vi "Cross_roads.vi"() -> ()   [LabVIEW 2024, in "Road.lvlib"]
uses:
  Road.lvlib
  typedef_GREEN.ctl
  typedef_YELLOW.ctl
  typedef_RED.ctl
  Enum_state.ctl
  typedef_Dane.ctl
  typedef_enum_cykl.ctl
  typedef_Enum_Stan.ctl
  typdef_Timer_Cluster.ctl
  typedef_Time.ctl
  MessageHandler/#typedef_MessageCommand.ctl
  MessageHandler/#typedef_MessageParameters.ctl
  MessageHandler/#typedef_MessageEnum.ctl
  MessageHandler/#typedef_CommunicationModuleAction.ctl
  MessageHandler/#typedef_Message.ctl
  GUI.lvlib
panel:
  in  "Boolean":bool
  out "State_4":bool
  out "Stoper":u32
  out "C3":T1
  out "C2":T1
  out "CC":T2
  out "D3":T3
  out "D2":T3
  out "DD":T4
  out "BBB":T5
  out "AA":T6
  out "A2":T7
  in  "Stop":bool
  out "BB":T5
  out "AAA":T6
  out "CCC":T2
  out "DDD":T4
  out "D1":T3
  out "C4":T11
  out "C1":T1
  out "B2":T12
  out "B1":T13
  out "A3":T14
  out "A1":T7
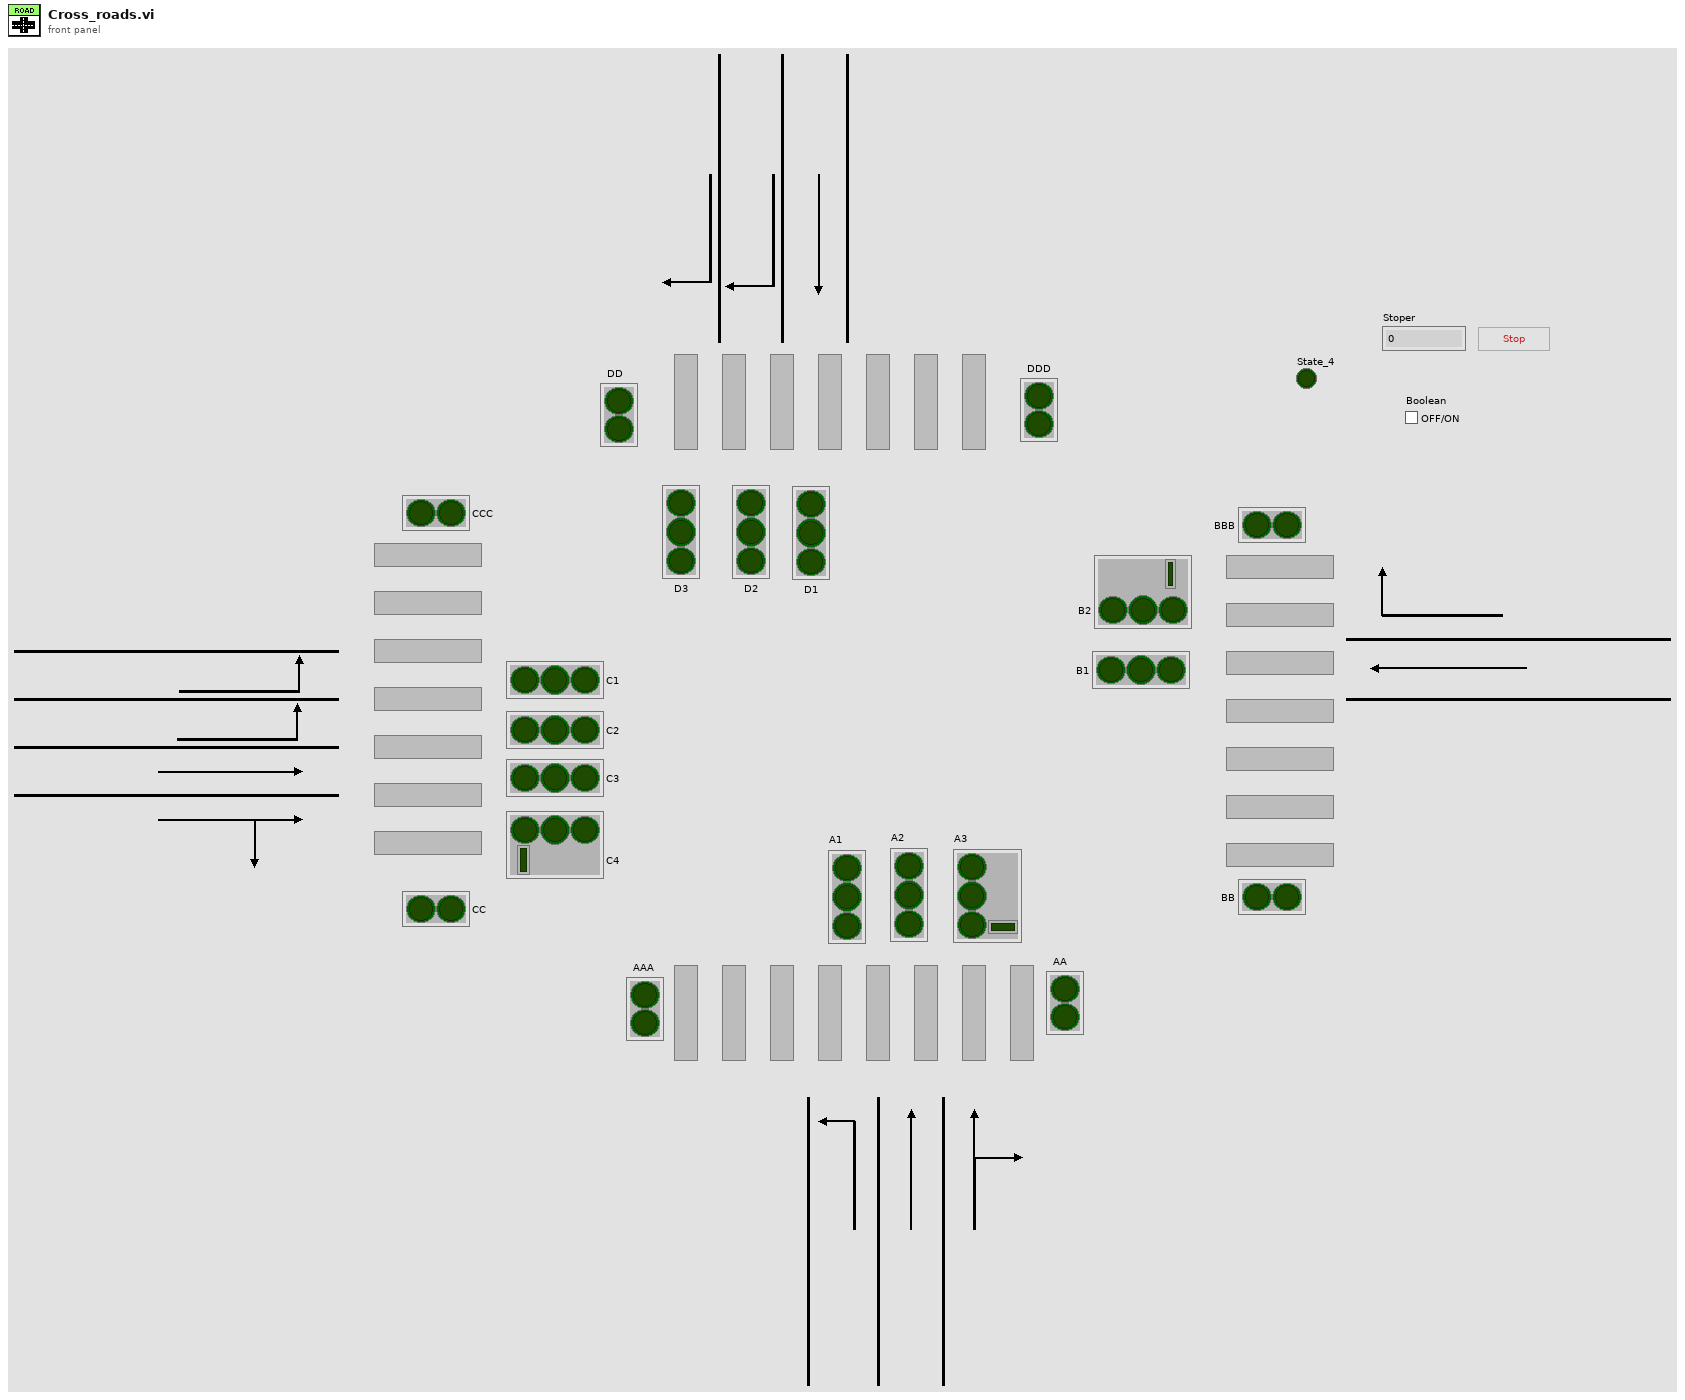
[diagram p1: front panel]
types:
  T1 = typedef "Road.lvlib/GUI.lvlib/typedef_Światła_C1.ctl" = cluster{"green":bool, "Yellow":bool, "red":bool}
  T2 = typedef "Road.lvlib/GUI.lvlib/typedef_Światła_CC.ctl" = cluster{"green":bool, "red":bool}
  T3 = typedef "Road.lvlib/GUI.lvlib/typedef_Światła_D1.ctl" = cluster{"green":bool, "Yellow":bool, "red":bool}
  T4 = typedef "Road.lvlib/GUI.lvlib/Światła_DD.ctl" = cluster{"green":bool, "red":bool}
  T5 = typedef "Road.lvlib/GUI.lvlib/typedef_Światła_BB.ctl" = cluster{"green":bool, "red":bool}
  T6 = typedef "Road.lvlib/GUI.lvlib/typdef_Światła_AA.ctl" = cluster{"green":bool, "red":bool}
  T7 = typedef "Road.lvlib/GUI.lvlib/typedef_Swiatła_A1.ctl" = cluster{"green":T8, "Yellow":T9, "red":T10}
  T8 = typedef "Road.lvlib/GUI.lvlib/typedef_GREEN.ctl" = bool
  T9 = typedef "Road.lvlib/GUI.lvlib/typedef_YELLOW.ctl" = bool
  T10 = typedef "Road.lvlib/GUI.lvlib/typedef_RED.ctl" = bool
  T11 = typedef "Road.lvlib/GUI.lvlib/typedef_Światła_C4.ctl" = cluster{"green":bool, "Yellow":bool, "red":bool, "Arrow":bool}
  T12 = typedef "Road.lvlib/GUI.lvlib/typdef_Światła_B2.ctl" = cluster{"green":bool, "Yellow":bool, "red":bool, "Arrow":bool}
  T13 = typedef "Road.lvlib/GUI.lvlib/typdef_Światła_B1.ctl" = cluster{"green":bool, "Yellow":bool, "red":bool}
  T14 = typedef "Road.lvlib/GUI.lvlib/typdef_Światła_A3.ctl" = cluster{"green":bool, "Yellow":bool, "red":bool, "Arrow":bool}
  T15 = typedef "Road.lvlib/GUI.lvlib/typedef_Dane.ctl" = cluster{"A1 ":T7, "A3":T14, "AAA":T6, "B1":T13, "B2":T12, "BBB":T5, "C1":T1, "C1 2":T1, "C4":T11, "CC":T2, "D1":T3, "D1 2":T3, "DD":T4, "A1  2":T7, "Enum_Cykl":T16, "Enum_Stan":T17, "Timer_Global":T18, "Timer_Mruganie":T18, "Time":T19, "Command":T20, "MessageParameters":T21}
  T16 = typedef "Road.lvlib/GUI.lvlib/typedef_enum_cykl.ctl" = enum16{"Init", "State_1", "State_2", "State_3", "State_4", "Breakdown"}
  T17 = typedef "Road.lvlib/GUI.lvlib/typedef_Enum_Stan.ctl" = enum16{"Czerwony", "Żółty", "Źielony", "Mruganie"}
  T18 = typedef "Road.lvlib/GUI.lvlib/typdef_Timer_Cluster.ctl" = cluster{"Numeric 3":u32, "Numeric 4":u32}
  T19 = typedef "Road.lvlib/GUI.lvlib/typedef_Time.ctl" = u32
  T20 = typedef "Road.lvlib/GUI.lvlib/#typedef_MessageCommand.ctl" = enum16{"CheckStatus", "NewData", "ShutDown"}
  T21 = typedef "Road.lvlib/GUI.lvlib/#typedef_MessageParameters.ctl" = cluster{"Status":T22, "Data":dbl[]}
  T22 = typedef "#typedef_MessageEnum.ctl" = enum16{"Light_ON", "IDLE", "Brakdown_ON", "Breakdown_OFF"}
  T23 = typedef "Road.lvlib/GUI.lvlib/Enum_state.ctl" = enum16{"Recive_data", "GUI_refresh", "Initialize", "Exit", "Send_data"}
  T24 = typedef "Road.lvlib/GUI.lvlib/#typedef_CommunicationModuleAction.ctl" = enum16{"ERROR_UnderRange", "Init", "Connect To existing", "Send Msg", "Priority Send", "Receive Msg", "Preview Messages", "ErrorHandle", "ShutDown", "ERROR_OverRange"}
  T25 = typedef "Road.lvlib/GUI.lvlib/#typedef_Message.ctl" = cluster{"Command":T20, "Parameters":T21}
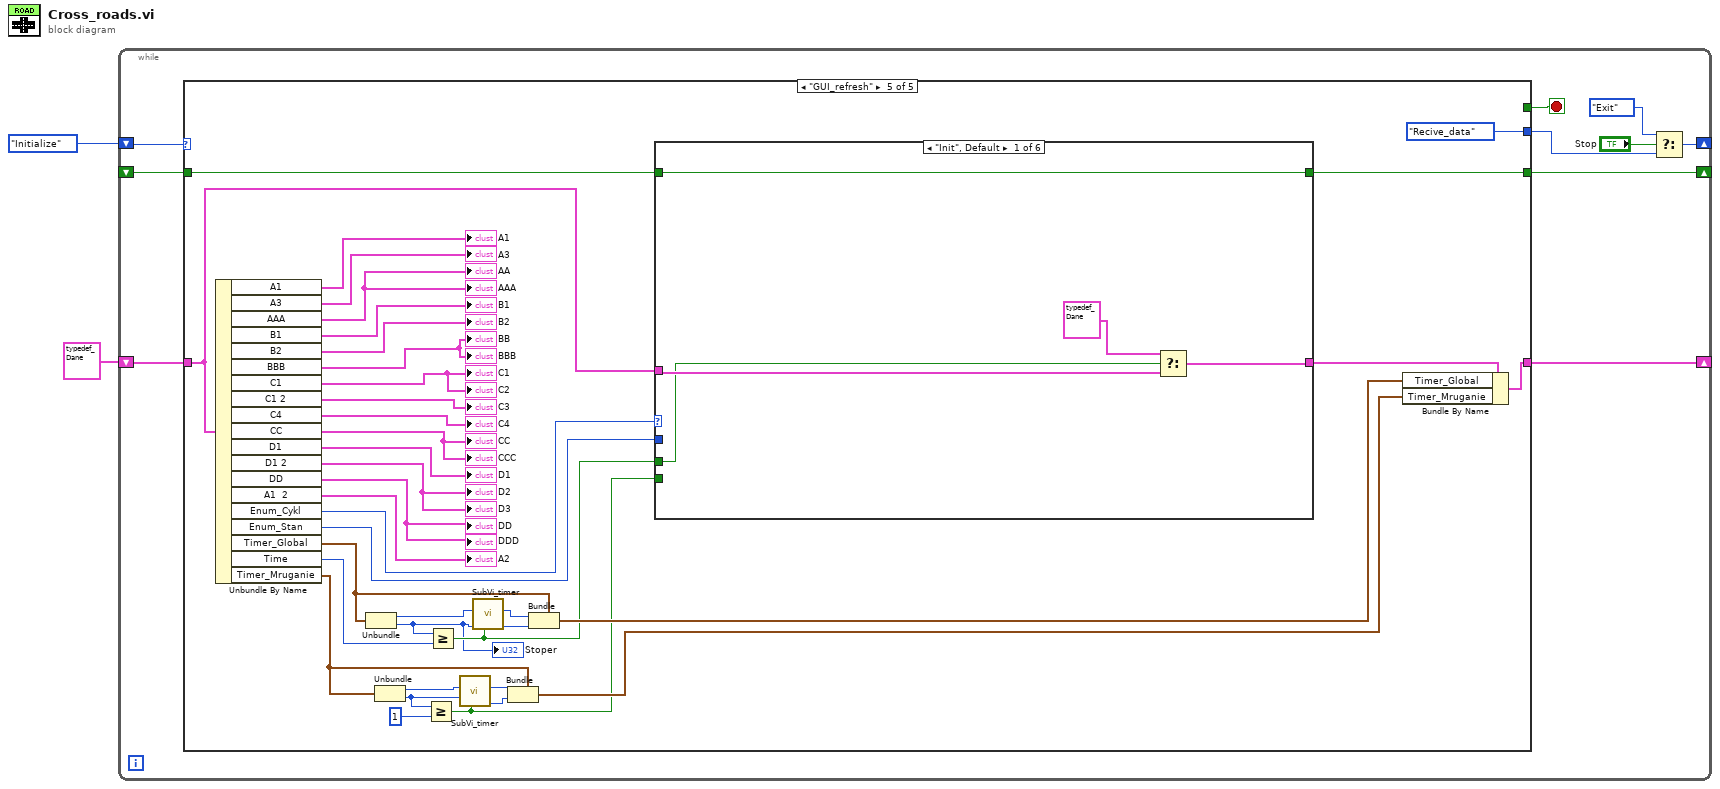
[diagram p0: block diagram]
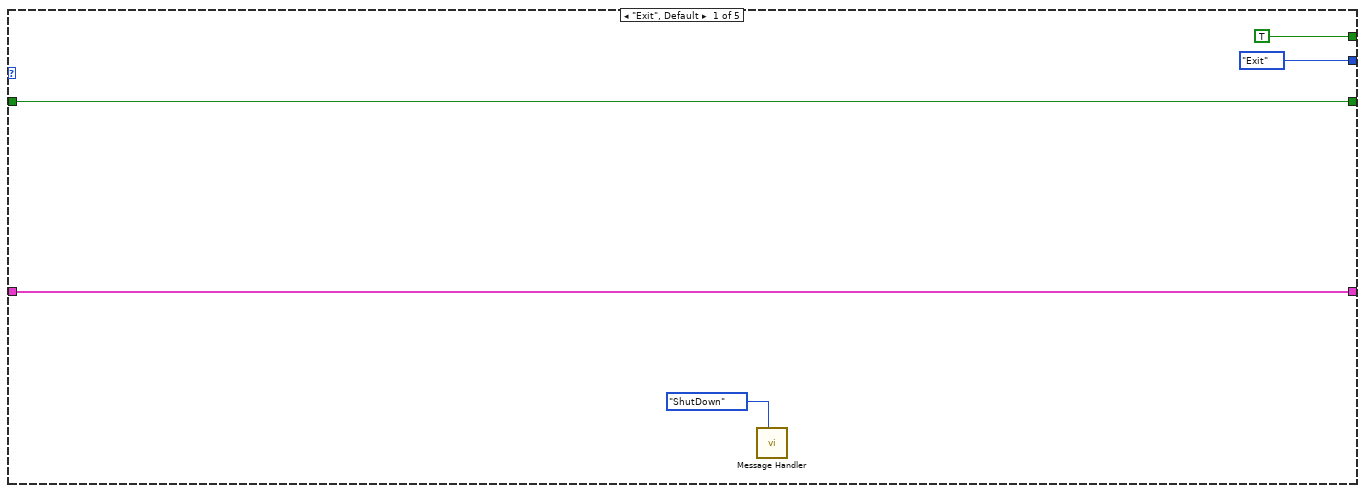
[diagram p2: hidden frame]
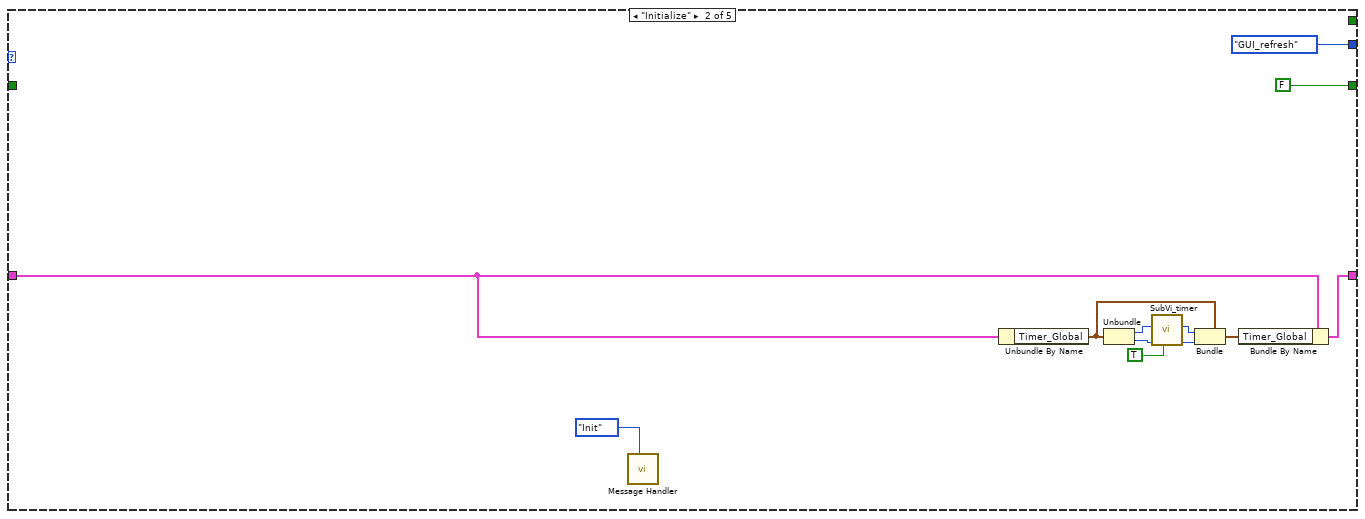
[diagram p3: hidden frame]
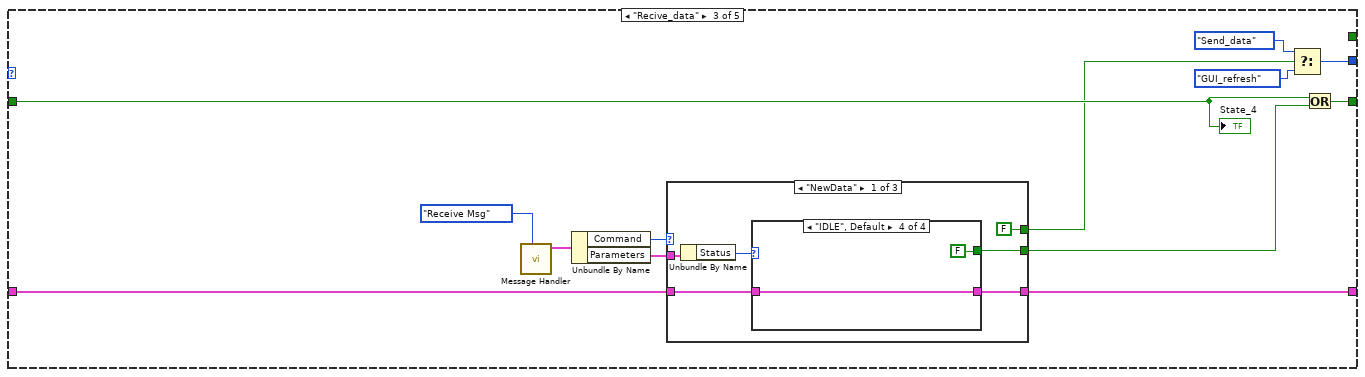
[diagram p4: hidden frame]
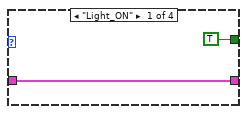
[diagram p5: hidden frame]
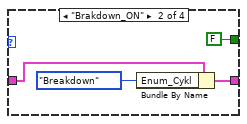
[diagram p6: hidden frame]
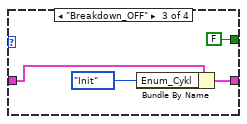
[diagram p7: hidden frame]
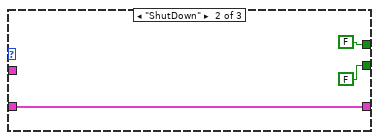
[diagram p8: hidden frame]
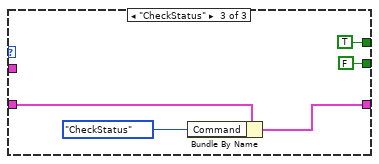
[diagram p9: hidden frame]
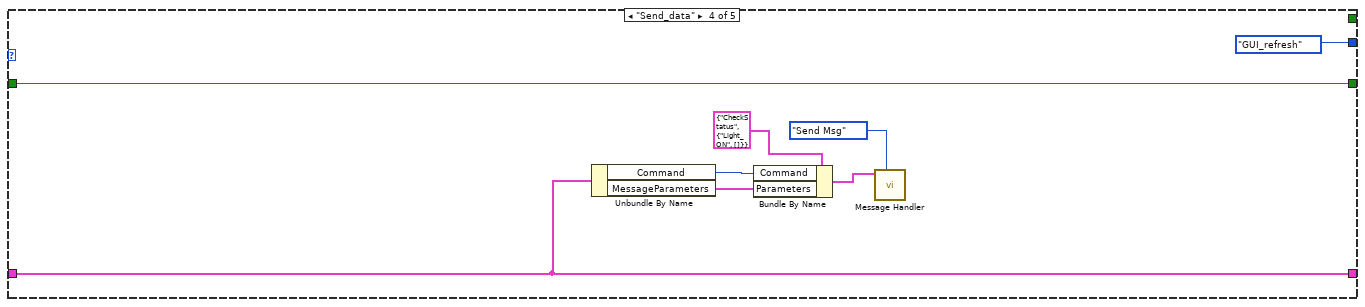
[diagram p10: hidden frame]
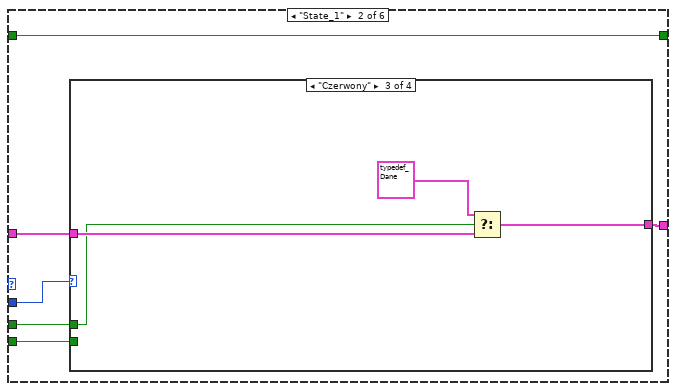
[diagram p11: hidden frame]
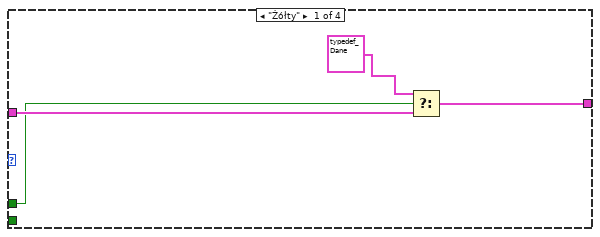
[diagram p12: hidden frame]
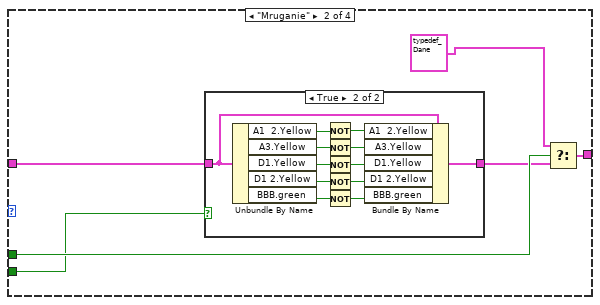
[diagram p13: hidden frame]
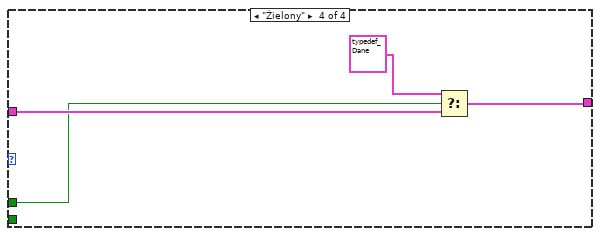
[diagram p15: hidden frame]
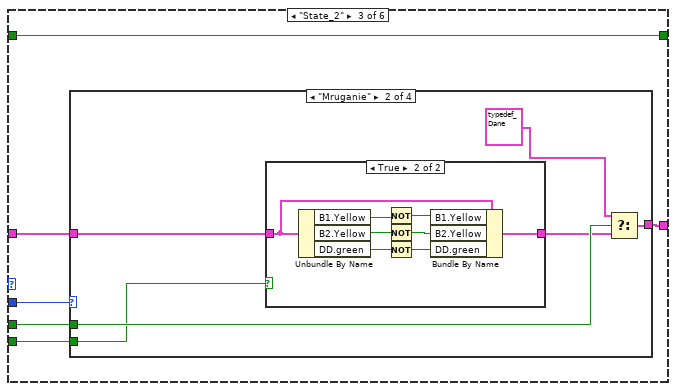
[diagram p16: hidden frame]
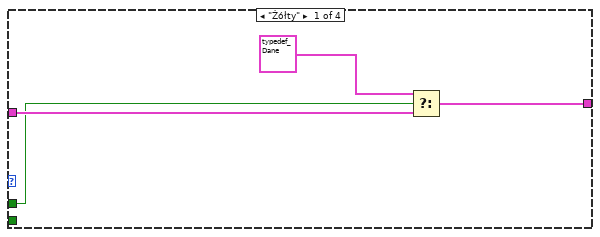
[diagram p17: hidden frame]
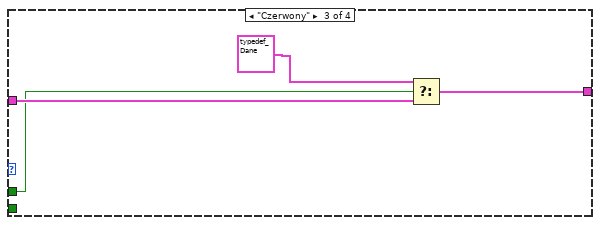
[diagram p19: hidden frame]
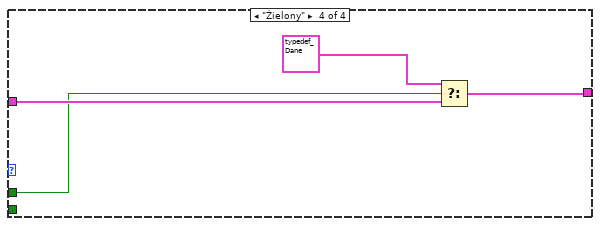
[diagram p20: hidden frame]
diagram:
  n1 = while {
    shift-right: [w11] -> _
    shift-left: Enum_state."Initialize" ("Enum") -> [w12]
    shift-right: [w5] -> _
    shift-left: T15 {"A1 "={"green"=TRUE, "Yellow"=TRUE, "red"=TRUE}, "A3"={"green"=TRUE, "Yellow"=TRUE, "red"=TRUE, "Arrow"=TRUE}, "AAA"={"green"=TRUE, "red"=TRUE}, "B1"={"green"=TRUE, "Yellow"=TRUE, "red"=TRUE}, "B2"={"green"=TRUE, "Yellow"=TRUE, "red"=TRUE, "Arrow"=TRUE}, "BBB"={"green"=TRUE, "red"=TRUE}, "C1"={"green"=TRUE, "Yellow"=TRUE, "red"=TRUE}, "C1 2"={"green"=TRUE, "Yellow"=TRUE, "red"=TRUE}, "C4"={"green"=TRUE, "Yellow"=TRUE, "red"=TRUE, "Arrow"=TRUE}, "CC"={"green"=TRUE, "red"=TRUE}, "D1"={"green"=TRUE, "Yellow"=TRUE, "red"=TRUE}, "D1 2"={"green"=TRUE, "Yellow"=TRUE, "red"=TRUE}, "DD"={"green"=TRUE, "red"=TRUE}, "A1  2"={"green"=TRUE, "Yellow"=TRUE, "red"=TRUE}, "Enum_Cykl"=enum."Init", "Enum_Stan"=enum."Czerwony", "Timer_Global"={"Numeric 3"=0, "Numeric 4"=0}, "Timer_Mruganie"={"Numeric 3"=0, "Numeric 4"=0}, "Time"=5, "Command"=enum."CheckStatus", "MessageParameters"={"Status"=enum."Light_ON", "Data"=[]}} -> [w6]
    shift-right: [w3] -> _
    shift-left: _ -> [w4]
    stop <- w8 stop-if-true
    n2 = case shown="\"GUI_refresh\"" w12 {
      tunnel: [Enum_state."Exit" Enum_state."GUI_refresh" ("Enum") w32 Enum_state."GUI_refresh" ("Enum") Enum_state."Recive_data" ("Enum")] -> w7
      tunnel: [TRUE _ _ _ _] -> w8
      tunnel: w6 -> [w15 w22 w31 w71 w113]
      tunnel: [w15 w23 w30 w71 w108] -> w5
      tunnel: w4 -> [w14 _ w42 w74 w78]
      tunnel: [w14 FALSE w41 w74 w77] -> w3
      frame "Exit", Default {
        n3 = call "Message Handler.vi"("Action"=#typedef_CommunicationModuleAction."ShutDown") -> ()  [unwired: 8 in, 3 out]
      }
      frame "Initialize" {
        n4 = call "Message Handler.vi"("Action"=#typedef_CommunicationModuleAction."Init") -> ()  [unwired: 8 in, 3 out]
        n5 = Unbundle By Name(w22) -> ("Timer_Global"=w24:T18)
        n6 = Unbundle(w24) -> ("Numeric 3"=w26:u32, "Numeric 4"=w21:u32)
        n7 = call "SubVi_timer.vi"("stop"=TRUE, "Numeric 2"=w21, "Numeric"=w26) -> ("Numeric 4"=w27:u32, "Numeric 3"=w28:u32)  [unwired: 7 in]
        n8 = Bundle(cluster=w24, "Numeric 3"=w28, "Numeric 4"=w27) -> (w25:T18)
        n9 = Bundle By Name(cluster=w22, "Timer_Global"=w25) -> (w23:T15)
      }
      frame "Recive_data" {
        n10 = call "Message Handler.vi"("Action"=#typedef_CommunicationModuleAction."Receive Msg") -> ("Message Out"=w39:T25)  [unwired: 8 in, 2 out]
        n11 = Unbundle By Name(w39) -> ("Command"=w38:T20, "Parameters"=w37:T21)
        n12 = case shown="\"NewData\"" w38 {
          tunnel: w37 -> [w48 _ _]
          tunnel: [w46 FALSE FALSE] -> w36
          tunnel: [FALSE FALSE TRUE] -> w35
          tunnel: w31 -> [w44 w61 w66]
          tunnel: [w43 w61 w65] -> w30
          frame "NewData" {
            n13 = Unbundle By Name(w48) -> ("Status"=w47:T22)
            n14 = case shown="\"IDLE\", Default" w47 {
              tunnel: [TRUE FALSE FALSE FALSE] -> w46
              tunnel: w44 -> [w49 w54 w58 w59]
              tunnel: [w49 w52 w56 w59] -> w43
              frame "Light_ON" {
              }
              frame "Brakdown_ON" {
                n15 = Bundle By Name(cluster=w54, "Enum_Cykl"=typedef_enum_cykl."Breakdown") -> (w52:T15)
              }
              frame "Breakdown_OFF" {
                n16 = Bundle By Name(cluster=w58, "Enum_Cykl"=typedef_enum_cykl."Init") -> (w56:T15)
              }
              frame "IDLE", Default {
              }
            }
          }
          frame "ShutDown" {
          }
          frame "CheckStatus" {
            n17 = Bundle By Name(cluster=w66, "Command"=#typedef_MessageCommand."CheckStatus") -> (w65:T15)
          }
        }
        n18 = Select(t=Enum_state."Send_data" ("Enum"), s=w35, f=Enum_state."GUI_refresh" ("Enum")) -> (s? t:f=w32:T23)
        n19 = Or(x=w42, y=w36) -> (x .or. y?=w41:bool)
        "State_4" <- w42
      }
      frame "Send_data" {
        n20 = Unbundle By Name(w71) -> ("Command"=w70:T20, "MessageParameters"=w69:T21)
        n21 = Bundle By Name(cluster=T25 {"Command"=enum."CheckStatus", "Parameters"={"Status"=enum."Light_ON", "Data"=[]}} ("Message"), "Command"=w70, "Parameters"=w69) -> (w72:T25)
        n22 = call "Message Handler.vi"("Action"=#typedef_CommunicationModuleAction."Send Msg", "Message"=w72) -> ()  [unwired: 7 in, 3 out]
      }
      frame "GUI_refresh" {
        n23 = Unbundle By Name(w113) -> ("A1"=→"A1":T7, "A3"=→"A3":T14, "AAA"=→"AAA" →"AA":T6, "B1"=→"B1":T13, "B2"=→"B2":T12, "BBB"=→"BB" →"BBB":T5, "C1"=→"C1" →"C2":T1, "C1 2"=→"C3":T1, "C4"=→"C4":T11, "CC"=→"CCC" →"CC":T2, "D1"=→"D1":T3, "D1 2"=→"D2" →"D3":T3, "DD"=→"DDD" →"DD":T4, "A1  2"=→"A2":T7, "Enum_Cykl"=w114:T16, "Enum_Stan"=w111:T17, "Timer_Global"=w90:T18, "Time"=w105:T19, "Timer_Mruganie"=w81:T18)
        n24 = Unbundle(w90) -> ("Numeric 3"=w112:u32, "Numeric 4"=w88:u32)
        "Stoper" <- w88
        n25 = Unbundle(w81) -> ("Numeric 3"=w86:u32, "Numeric 4"=w85:u32)
        n26 = Greater Or Equal?(x=w85, y=u32 1) -> (x >= y?=w80:bool)
        n27 = Greater Or Equal?(x=w88, y=w105) -> (x >= y?=w104:bool)
        n28 = call "SubVi_timer.vi"("stop"=w80, "Numeric 2"=w85, "Numeric"=w86) -> ("Numeric 4"=w83:u32, "Numeric 3"=w84:u32)  [unwired: 7 in]
        n29 = call "SubVi_timer.vi"("stop"=w104, "Numeric 2"=w88, "Numeric"=w112) -> ("Numeric 4"=w89:u32, "Numeric 3"=w106:u32)  [unwired: 7 in]
        n30 = Bundle(cluster=w81, "Numeric 3"=w84, "Numeric 4"=w83) -> (w82:T18)
        n31 = Bundle(cluster=w90, "Numeric 3"=w106, "Numeric 4"=w89) -> (w107:T18)
        n32 = case shown="\"Init\", Default" w114 {
          tunnel: [w118 w125 w162 w195 w233 w263] -> w109
          tunnel: w104 -> [w116 w124 w161 w194 w232 _]
          tunnel: w113 -> [w117 w123 w160 w193 w231 _]
          tunnel: w111 -> [_ w122 w159 w192 w230 _]
          tunnel: w80 -> [_ w121 w158 w191 w229 w265]
          tunnel: w78 -> [w115 w120 w157 w190 _ w266]
          tunnel: [w115 w120 w157 w190 FALSE w266] -> w77
          frame "Init", Default {
            n33 = Select(t=T15 {"A1 "={"green"=FALSE, "Yellow"=FALSE, "red"=TRUE}, "A3"={"green"=FALSE, "Yellow"=FALSE, "red"=TRUE, "Arrow"=FALSE}, "AAA"={"green"=FALSE, "red"=TRUE}, "B1"={"green"=FALSE, "Yellow"=FALSE, "red"=TRUE}, "B2"={"green"=FALSE, "Yellow"=FALSE, "red"=TRUE, "Arrow"=FALSE}, "BBB"={"green"=FALSE, "red"=TRUE}, "C1"={"green"=FALSE, "Yellow"=FALSE, "red"=TRUE}, "C1 2"={"green"=FALSE, "Yellow"=FALSE, "red"=TRUE}, "C4"={"green"=FALSE, "Yellow"=FALSE, "red"=TRUE, "Arrow"=FALSE}, "CC"={"green"=FALSE, "red"=TRUE}, "D1"={"green"=FALSE, "Yellow"=FALSE, "red"=TRUE}, "D1 2"={"green"=FALSE, "Yellow"=FALSE, "red"=TRUE}, "DD"={"green"=FALSE, "red"=TRUE}, "A1  2"={"green"=FALSE, "Yellow"=FALSE, "red"=TRUE}, "Enum_Cykl"=enum."State_1", "Enum_Stan"=enum."Czerwony", "Timer_Global"={"Numeric 3"=0, "Numeric 4"=0}, "Timer_Mruganie"={"Numeric 3"=0, "Numeric 4"=0}, "Time"=2, "Command"=enum."CheckStatus", "MessageParameters"={"Status"=enum."Light_ON", "Data"=[]}}, s=w116, f=w117) -> (s? t:f=w118:T15)
          }
          frame "State_1" {
            n34 = case shown="\"Czerwony\"" w122 {
              tunnel: [w127 w134 w150 w155] -> w125
              tunnel: w124 -> [w128 w135 w151 w153]
              tunnel: w123 -> [w129 w133 w152 w156]
              tunnel: w121 -> [_ w131 _ _]
              frame "Żółty" {
                n35 = Select(t=T15 {"A1 "={"green"=FALSE, "Yellow"=FALSE, "red"=TRUE}, "A3"={"green"=TRUE, "Yellow"=FALSE, "red"=FALSE, "Arrow"=FALSE}, "AAA"={"green"=FALSE, "red"=TRUE}, "B1"={"green"=FALSE, "Yellow"=FALSE, "red"=TRUE}, "B2"={"green"=FALSE, "Yellow"=FALSE, "red"=TRUE, "Arrow"=TRUE}, "BBB"={"green"=TRUE, "red"=FALSE}, "C1"={"green"=FALSE, "Yellow"=FALSE, "red"=TRUE}, "C1 2"={"green"=FALSE, "Yellow"=FALSE, "red"=TRUE}, "C4"={"green"=FALSE, "Yellow"=FALSE, "red"=TRUE, "Arrow"=TRUE}, "CC"={"green"=FALSE, "red"=TRUE}, "D1"={"green"=TRUE, "Yellow"=FALSE, "red"=FALSE}, "D1 2"={"green"=TRUE, "Yellow"=FALSE, "red"=FALSE}, "DD"={"green"=FALSE, "red"=TRUE}, "A1  2"={"green"=TRUE, "Yellow"=FALSE, "red"=FALSE}, "Enum_Cykl"=enum."State_1", "Enum_Stan"=enum."Źielony", "Timer_Global"={"Numeric 3"=0, "Numeric 4"=0}, "Timer_Mruganie"={"Numeric 3"=0, "Numeric 4"=0}, "Time"=3, "Command"=enum."CheckStatus", "MessageParameters"={"Status"=enum."Light_ON", "Data"=[]}}, s=w128, f=w129) -> (s? t:f=w127:T15)
              }
              frame "Mruganie" {
                n36 = case shown="True" w131 {
                  tunnel: [w136 w137] -> w132
                  tunnel: w133 -> [w136 w138]
                  frame False {
                  }
                  frame True {
                    n37 = Unbundle By Name(w138) -> ("A1  2.Yellow"=w147:T9, "A3.Yellow"=w148:bool, "D1.Yellow"=w146:bool, "D1 2.Yellow"=w145:bool, "BBB.green"=w144:bool)
                    n38 = Not(x=w147) -> (.not. x?=w143:T9)
                    n39 = Not(x=w148) -> (.not. x?=w142:bool)
                    n40 = Not(x=w146) -> (.not. x?=w141:bool)
                    n41 = Not(x=w145) -> (.not. x?=w140:bool)
                    n42 = Not(x=w144) -> (.not. x?=w139:bool)
                    n43 = Bundle By Name(cluster=w138, "A1  2.Yellow"=w143, "A3.Yellow"=w142, "D1.Yellow"=w141, "D1 2.Yellow"=w140, "BBB.green"=w139) -> (w137:T15)
                  }
                }
                n44 = Select(t=T15 {"A1 "={"green"=FALSE, "Yellow"=FALSE, "red"=TRUE}, "A3"={"green"=FALSE, "Yellow"=FALSE, "red"=TRUE, "Arrow"=FALSE}, "AAA"={"green"=FALSE, "red"=TRUE}, "B1"={"green"=FALSE, "Yellow"=FALSE, "red"=TRUE}, "B2"={"green"=FALSE, "Yellow"=FALSE, "red"=TRUE, "Arrow"=FALSE}, "BBB"={"green"=FALSE, "red"=TRUE}, "C1"={"green"=FALSE, "Yellow"=FALSE, "red"=TRUE}, "C1 2"={"green"=FALSE, "Yellow"=FALSE, "red"=TRUE}, "C4"={"green"=FALSE, "Yellow"=FALSE, "red"=TRUE, "Arrow"=FALSE}, "CC"={"green"=FALSE, "red"=TRUE}, "D1"={"green"=FALSE, "Yellow"=FALSE, "red"=TRUE}, "D1 2"={"green"=FALSE, "Yellow"=FALSE, "red"=TRUE}, "DD"={"green"=FALSE, "red"=TRUE}, "A1  2"={"green"=FALSE, "Yellow"=FALSE, "red"=TRUE}, "Enum_Cykl"=enum."State_2", "Enum_Stan"=enum."Czerwony", "Timer_Global"={"Numeric 3"=0, "Numeric 4"=0}, "Timer_Mruganie"={"Numeric 3"=0, "Numeric 4"=0}, "Time"=2, "Command"=enum."CheckStatus", "MessageParameters"={"Status"=enum."Light_ON", "Data"=[]}}, s=w135, f=w132) -> (s? t:f=w134:T15)
              }
              frame "Czerwony" {
                n45 = Select(t=T15 {"A1 "={"green"=FALSE, "Yellow"=FALSE, "red"=TRUE}, "A3"={"green"=FALSE, "Yellow"=TRUE, "red"=TRUE, "Arrow"=FALSE}, "AAA"={"green"=FALSE, "red"=TRUE}, "B1"={"green"=FALSE, "Yellow"=FALSE, "red"=TRUE}, "B2"={"green"=FALSE, "Yellow"=FALSE, "red"=TRUE, "Arrow"=FALSE}, "BBB"={"green"=FALSE, "red"=TRUE}, "C1"={"green"=FALSE, "Yellow"=FALSE, "red"=TRUE}, "C1 2"={"green"=FALSE, "Yellow"=FALSE, "red"=TRUE}, "C4"={"green"=FALSE, "Yellow"=FALSE, "red"=TRUE, "Arrow"=FALSE}, "CC"={"green"=FALSE, "red"=TRUE}, "D1"={"green"=FALSE, "Yellow"=TRUE, "red"=TRUE}, "D1 2"={"green"=FALSE, "Yellow"=TRUE, "red"=TRUE}, "DD"={"green"=FALSE, "red"=TRUE}, "A1  2"={"green"=FALSE, "Yellow"=TRUE, "red"=TRUE}, "Enum_Cykl"=enum."State_1", "Enum_Stan"=enum."Żółty", "Timer_Global"={"Numeric 3"=0, "Numeric 4"=0}, "Timer_Mruganie"={"Numeric 3"=0, "Numeric 4"=0}, "Time"=3, "Command"=enum."CheckStatus", "MessageParameters"={"Status"=enum."Light_ON", "Data"=[]}}, s=w151, f=w152) -> (s? t:f=w150:T15)
              }
              frame "Źielony" {
                n46 = Select(t=T15 {"A1 "={"green"=FALSE, "Yellow"=FALSE, "red"=TRUE}, "A3"={"green"=FALSE, "Yellow"=TRUE, "red"=FALSE, "Arrow"=FALSE}, "AAA"={"green"=FALSE, "red"=TRUE}, "B1"={"green"=FALSE, "Yellow"=FALSE, "red"=TRUE}, "B2"={"green"=FALSE, "Yellow"=FALSE, "red"=TRUE, "Arrow"=FALSE}, "BBB"={"green"=TRUE, "red"=FALSE}, "C1"={"green"=FALSE, "Yellow"=FALSE, "red"=TRUE}, "C1 2"={"green"=FALSE, "Yellow"=FALSE, "red"=TRUE}, "C4"={"green"=FALSE, "Yellow"=FALSE, "red"=TRUE, "Arrow"=FALSE}, "CC"={"green"=FALSE, "red"=TRUE}, "D1"={"green"=FALSE, "Yellow"=TRUE, "red"=FALSE}, "D1 2"={"green"=FALSE, "Yellow"=TRUE, "red"=FALSE}, "DD"={"green"=FALSE, "red"=TRUE}, "A1  2"={"green"=FALSE, "Yellow"=TRUE, "red"=FALSE}, "Enum_Cykl"=enum."State_1", "Enum_Stan"=enum."Mruganie", "Timer_Global"={"Numeric 3"=0, "Numeric 4"=0}, "Timer_Mruganie"={"Numeric 3"=0, "Numeric 4"=0}, "Time"=5, "Command"=enum."CheckStatus", "MessageParameters"={"Status"=enum."Light_ON", "Data"=[]}}, s=w153, f=w156) -> (s? t:f=w155:T15)
              }
            }
          }
          frame "State_2" {
            n47 = case shown="\"Mruganie\"" w159 {
              tunnel: [w164 w171 w183 w188] -> w162
              tunnel: w161 -> [w165 w172 w184 w187]
              tunnel: w160 -> [w166 w170 w185 w189]
              tunnel: w158 -> [_ w168 _ _]
              frame "Żółty" {
                n48 = Select(t=T15 {"A1 "={"green"=FALSE, "Yellow"=FALSE, "red"=TRUE}, "A3"={"green"=FALSE, "Yellow"=FALSE, "red"=TRUE, "Arrow"=FALSE}, "AAA"={"green"=TRUE, "red"=FALSE}, "B1"={"green"=TRUE, "Yellow"=FALSE, "red"=FALSE}, "B2"={"green"=TRUE, "Yellow"=FALSE, "red"=FALSE, "Arrow"=FALSE}, "BBB"={"green"=FALSE, "red"=TRUE}, "C1"={"green"=FALSE, "Yellow"=FALSE, "red"=TRUE}, "C1 2"={"green"=TRUE, "Yellow"=FALSE, "red"=FALSE}, "C4"={"green"=TRUE, "Yellow"=FALSE, "red"=FALSE, "Arrow"=FALSE}, "CC"={"green"=FALSE, "red"=TRUE}, "D1"={"green"=FALSE, "Yellow"=FALSE, "red"=TRUE}, "D1 2"={"green"=FALSE, "Yellow"=FALSE, "red"=TRUE}, "DD"={"green"=TRUE, "red"=FALSE}, "A1  2"={"green"=FALSE, "Yellow"=FALSE, "red"=TRUE}, "Enum_Cykl"=enum."State_2", "Enum_Stan"=enum."Źielony", "Timer_Global"={"Numeric 3"=0, "Numeric 4"=0}, "Timer_Mruganie"={"Numeric 3"=0, "Numeric 4"=0}, "Time"=3, "Command"=enum."CheckStatus", "MessageParameters"={"Status"=enum."Light_ON", "Data"=[]}}, s=w165, f=w166) -> (s? t:f=w164:T15)
              }
              frame "Mruganie" {
                n49 = case shown="True" w168 {
                  tunnel: [w173 w174] -> w169
                  tunnel: w170 -> [w173 w175]
                  frame False {
                  }
                  frame True {
                    n50 = Unbundle By Name(w175) -> ("B1.Yellow"=w180:bool, "B2.Yellow"=w181:bool, "DD.green"=w179:bool)
                    n51 = Not(x=w180) -> (.not. x?=w178:bool)
                    n52 = Not(x=w181) -> (.not. x?=w177:bool)
                    n53 = Not(x=w179) -> (.not. x?=w176:bool)
                    n54 = Bundle By Name(cluster=w175, "B1.Yellow"=w178, "B2.Yellow"=w177, "DD.green"=w176) -> (w174:T15)
                  }
                }
                n55 = Select(t=T15 {"A1 "={"green"=FALSE, "Yellow"=FALSE, "red"=TRUE}, "A3"={"green"=FALSE, "Yellow"=FALSE, "red"=TRUE, "Arrow"=FALSE}, "AAA"={"green"=TRUE, "red"=FALSE}, "B1"={"green"=FALSE, "Yellow"=FALSE, "red"=TRUE}, "B2"={"green"=FALSE, "Yellow"=FALSE, "red"=TRUE, "Arrow"=FALSE}, "BBB"={"green"=FALSE, "red"=TRUE}, "C1"={"green"=FALSE, "Yellow"=TRUE, "red"=TRUE}, "C1 2"={"green"=TRUE, "Yellow"=FALSE, "red"=FALSE}, "C4"={"green"=TRUE, "Yellow"=FALSE, "red"=FALSE, "Arrow"=FALSE}, "CC"={"green"=FALSE, "red"=TRUE}, "D1"={"green"=FALSE, "Yellow"=FALSE, "red"=TRUE}, "D1 2"={"green"=FALSE, "Yellow"=FALSE, "red"=TRUE}, "DD"={"green"=FALSE, "red"=TRUE}, "A1  2"={"green"=FALSE, "Yellow"=FALSE, "red"=TRUE}, "Enum_Cykl"=enum."State_3", "Enum_Stan"=enum."Żółty", "Timer_Global"={"Numeric 3"=0, "Numeric 4"=0}, "Timer_Mruganie"={"Numeric 3"=0, "Numeric 4"=0}, "Time"=3, "Command"=enum."CheckStatus", "MessageParameters"={"Status"=enum."Light_ON", "Data"=[]}}, s=w172, f=w169) -> (s? t:f=w171:T15)
              }
              frame "Czerwony" {
                n56 = Select(t=T15 {"A1 "={"green"=FALSE, "Yellow"=FALSE, "red"=TRUE}, "A3"={"green"=FALSE, "Yellow"=FALSE, "red"=TRUE, "Arrow"=FALSE}, "AAA"={"green"=FALSE, "red"=TRUE}, "B1"={"green"=FALSE, "Yellow"=TRUE, "red"=TRUE}, "B2"={"green"=FALSE, "Yellow"=TRUE, "red"=TRUE, "Arrow"=FALSE}, "BBB"={"green"=FALSE, "red"=TRUE}, "C1"={"green"=FALSE, "Yellow"=FALSE, "red"=TRUE}, "C1 2"={"green"=FALSE, "Yellow"=TRUE, "red"=TRUE}, "C4"={"green"=FALSE, "Yellow"=TRUE, "red"=TRUE, "Arrow"=FALSE}, "CC"={"green"=FALSE, "red"=TRUE}, "D1"={"green"=FALSE, "Yellow"=FALSE, "red"=TRUE}, "D1 2"={"green"=FALSE, "Yellow"=FALSE, "red"=TRUE}, "DD"={"green"=FALSE, "red"=TRUE}, "A1  2"={"green"=FALSE, "Yellow"=FALSE, "red"=TRUE}, "Enum_Cykl"=enum."State_2", "Enum_Stan"=enum."Żółty", "Timer_Global"={"Numeric 3"=0, "Numeric 4"=0}, "Timer_Mruganie"={"Numeric 3"=0, "Numeric 4"=0}, "Time"=3, "Command"=enum."CheckStatus", "MessageParameters"={"Status"=enum."Light_ON", "Data"=[]}}, s=w184, f=w185) -> (s? t:f=w183:T15)
              }
              frame "Źielony" {
                n57 = Select(t=T15 {"A1 "={"green"=FALSE, "Yellow"=FALSE, "red"=TRUE}, "A3"={"green"=FALSE, "Yellow"=FALSE, "red"=TRUE, "Arrow"=FALSE}, "AAA"={"green"=TRUE, "red"=FALSE}, "B1"={"green"=FALSE, "Yellow"=TRUE, "red"=FALSE}, "B2"={"green"=FALSE, "Yellow"=TRUE, "red"=FALSE, "Arrow"=FALSE}, "BBB"={"green"=FALSE, "red"=TRUE}, "C1"={"green"=FALSE, "Yellow"=FALSE, "red"=TRUE}, "C1 2"={"green"=TRUE, "Yellow"=FALSE, "red"=FALSE}, "C4"={"green"=TRUE, "Yellow"=FALSE, "red"=FALSE, "Arrow"=FALSE}, "CC"={"green"=FALSE, "red"=TRUE}, "D1"={"green"=FALSE, "Yellow"=FALSE, "red"=TRUE}, "D1 2"={"green"=FALSE, "Yellow"=FALSE, "red"=TRUE}, "DD"={"green"=TRUE, "red"=FALSE}, "A1  2"={"green"=FALSE, "Yellow"=FALSE, "red"=TRUE}, "Enum_Cykl"=enum."State_2", "Enum_Stan"=enum."Mruganie", "Timer_Global"={"Numeric 3"=0, "Numeric 4"=0}, "Timer_Mruganie"={"Numeric 3"=0, "Numeric 4"=0}, "Time"=3, "Command"=enum."CheckStatus", "MessageParameters"={"Status"=enum."Light_ON", "Data"=[]}}, s=w187, f=w189) -> (s? t:f=w188:T15)
              }
            }
          }
          frame "State_3" {
            n58 = case shown="\"Mruganie\"" w192 {
              tunnel: [w197 w201 w209 w226] -> w195
              tunnel: w194 -> [w198 w202 w210 w225]
              tunnel: w193 -> [w199 w203 w206 w227]
              tunnel: w191 -> [_ _ w207 _]
              tunnel: w190 -> [_ _ w204 _]
              frame "Żółty" {
                n59 = Select(t=T15 {"A1 "={"green"=FALSE, "Yellow"=FALSE, "red"=TRUE}, "A3"={"green"=FALSE, "Yellow"=FALSE, "red"=TRUE, "Arrow"=FALSE}, "AAA"={"green"=TRUE, "red"=FALSE}, "B1"={"green"=FALSE, "Yellow"=FALSE, "red"=TRUE}, "B2"={"green"=FALSE, "Yellow"=FALSE, "red"=TRUE, "Arrow"=FALSE}, "BBB"={"green"=FALSE, "red"=TRUE}, "C1"={"green"=TRUE, "Yellow"=FALSE, "red"=FALSE}, "C1 2"={"green"=TRUE, "Yellow"=FALSE, "red"=FALSE}, "C4"={"green"=TRUE, "Yellow"=FALSE, "red"=FALSE, "Arrow"=FALSE}, "CC"={"green"=FALSE, "red"=TRUE}, "D1"={"green"=FALSE, "Yellow"=FALSE, "red"=TRUE}, "D1 2"={"green"=FALSE, "Yellow"=FALSE, "red"=TRUE}, "DD"={"green"=FALSE, "red"=TRUE}, "A1  2"={"green"=FALSE, "Yellow"=FALSE, "red"=TRUE}, "Enum_Cykl"=enum."State_3", "Enum_Stan"=enum."Źielony", "Timer_Global"={"Numeric 3"=0, "Numeric 4"=0}, "Timer_Mruganie"={"Numeric 3"=0, "Numeric 4"=0}, "Time"=5, "Command"=enum."CheckStatus", "MessageParameters"={"Status"=enum."Light_ON", "Data"=[]}}, s=w198, f=w199) -> (s? t:f=w197:T15)
              }
              frame "Czerwony" {
                n60 = Select(t=T15 {"A1 "={"green"=FALSE, "Yellow"=FALSE, "red"=TRUE}, "A3"={"green"=FALSE, "Yellow"=FALSE, "red"=TRUE, "Arrow"=FALSE}, "AAA"={"green"=TRUE, "red"=FALSE}, "B1"={"green"=FALSE, "Yellow"=FALSE, "red"=TRUE}, "B2"={"green"=FALSE, "Yellow"=FALSE, "red"=TRUE, "Arrow"=FALSE}, "BBB"={"green"=FALSE, "red"=TRUE}, "C1"={"green"=TRUE, "Yellow"=FALSE, "red"=FALSE}, "C1 2"={"green"=TRUE, "Yellow"=FALSE, "red"=FALSE}, "C4"={"green"=TRUE, "Yellow"=FALSE, "red"=FALSE, "Arrow"=FALSE}, "CC"={"green"=FALSE, "red"=TRUE}, "D1"={"green"=FALSE, "Yellow"=FALSE, "red"=TRUE}, "D1 2"={"green"=FALSE, "Yellow"=FALSE, "red"=TRUE}, "DD"={"green"=FALSE, "red"=TRUE}, "A1  2"={"green"=FALSE, "Yellow"=FALSE, "red"=TRUE}, "Enum_Cykl"=enum."State_3", "Enum_Stan"=enum."Źielony", "Timer_Global"={"Numeric 3"=0, "Numeric 4"=0}, "Timer_Mruganie"={"Numeric 3"=0, "Numeric 4"=0}, "Time"=3, "Command"=enum."CheckStatus", "MessageParameters"={"Status"=enum."Light_ON", "Data"=[]}}, s=w202, f=w203) -> (s? t:f=w201:T15)
              }
              frame "Mruganie" {
                n61 = case shown="True" w207 {
                  tunnel: [w213 w214] -> w208
                  tunnel: w206 -> [w213 w215]
                  frame False {
                  }
                  frame True {
                    n62 = Unbundle By Name(w215) -> ("C1.Yellow"=w222:bool, "C1 2.Yellow"=w223:bool, "C4.Yellow"=w221:bool, "AAA.green"=w220:bool)
                    n63 = Not(x=w222) -> (.not. x?=w219:bool)
                    n64 = Not(x=w223) -> (.not. x?=w218:bool)
                    n65 = Not(x=w221) -> (.not. x?=w217:bool)
                    n66 = Not(x=w220) -> (.not. x?=w216:bool)
                    n67 = Bundle By Name(cluster=w215, "C1.Yellow"=w219, "C1 2.Yellow"=w218, "C4.Yellow"=w217, "AAA.green"=w216) -> (w214:T15)
                  }
                }
                n68 = case shown="True" w204 {
                  tunnel: [T15 {"A1 "={"green"=FALSE, "Yellow"=FALSE, "red"=TRUE}, "A3"={"green"=FALSE, "Yellow"=FALSE, "red"=TRUE, "Arrow"=FALSE}, "AAA"={"green"=FALSE, "red"=TRUE}, "B1"={"green"=FALSE, "Yellow"=FALSE, "red"=TRUE}, "B2"={"green"=FALSE, "Yellow"=FALSE, "red"=TRUE, "Arrow"=FALSE}, "BBB"={"green"=FALSE, "red"=TRUE}, "C1"={"green"=FALSE, "Yellow"=FALSE, "red"=TRUE}, "C1 2"={"green"=FALSE, "Yellow"=FALSE, "red"=TRUE}, "C4"={"green"=FALSE, "Yellow"=FALSE, "red"=TRUE, "Arrow"=FALSE}, "CC"={"green"=FALSE, "red"=TRUE}, "D1"={"green"=FALSE, "Yellow"=FALSE, "red"=TRUE}, "D1 2"={"green"=FALSE, "Yellow"=FALSE, "red"=TRUE}, "DD"={"green"=FALSE, "red"=TRUE}, "A1  2"={"green"=FALSE, "Yellow"=FALSE, "red"=TRUE}, "Enum_Cykl"=enum."State_1", "Enum_Stan"=enum."Czerwony", "Timer_Global"={"Numeric 3"=0, "Numeric 4"=0}, "Timer_Mruganie"={"Numeric 3"=0, "Numeric 4"=0}, "Time"=1, "Command"=enum."CheckStatus", "MessageParameters"={"Status"=enum."Light_ON", "Data"=[]}} T15 {"A1 "={"green"=FALSE, "Yellow"=FALSE, "red"=TRUE}, "A3"={"green"=FALSE, "Yellow"=FALSE, "red"=TRUE, "Arrow"=FALSE}, "AAA"={"green"=FALSE, "red"=TRUE}, "B1"={"green"=FALSE, "Yellow"=FALSE, "red"=TRUE}, "B2"={"green"=FALSE, "Yellow"=FALSE, "red"=TRUE, "Arrow"=FALSE}, "BBB"={"green"=FALSE, "red"=TRUE}, "C1"={"green"=FALSE, "Yellow"=FALSE, "red"=TRUE}, "C1 2"={"green"=FALSE, "Yellow"=FALSE, "red"=TRUE}, "C4"={"green"=FALSE, "Yellow"=FALSE, "red"=TRUE, "Arrow"=FALSE}, "CC"={"green"=FALSE, "red"=TRUE}, "D1"={"green"=FALSE, "Yellow"=FALSE, "red"=TRUE}, "D1 2"={"green"=FALSE, "Yellow"=FALSE, "red"=TRUE}, "DD"={"green"=FALSE, "red"=TRUE}, "A1  2"={"green"=FALSE, "Yellow"=FALSE, "red"=TRUE}, "Enum_Cykl"=enum."State_4", "Enum_Stan"=enum."Czerwony", "Timer_Global"={"Numeric 3"=0, "Numeric 4"=0}, "Timer_Mruganie"={"Numeric 3"=0, "Numeric 4"=0}, "Time"=1, "Command"=enum."CheckStatus", "MessageParameters"={"Status"=enum."Light_ON", "Data"=[]}}] -> w205
                  frame False {
                  }
                  frame True {
                  }
                }
                n69 = Select(t=w205, s=w210, f=w208) -> (s? t:f=w209:T15)
              }
              frame "Źielony" {
                n70 = Select(t=T15 {"A1 "={"green"=FALSE, "Yellow"=FALSE, "red"=TRUE}, "A3"={"green"=FALSE, "Yellow"=FALSE, "red"=TRUE, "Arrow"=FALSE}, "AAA"={"green"=TRUE, "red"=FALSE}, "B1"={"green"=FALSE, "Yellow"=FALSE, "red"=TRUE}, "B2"={"green"=FALSE, "Yellow"=FALSE, "red"=TRUE, "Arrow"=FALSE}, "BBB"={"green"=FALSE, "red"=TRUE}, "C1"={"green"=FALSE, "Yellow"=TRUE, "red"=FALSE}, "C1 2"={"green"=FALSE, "Yellow"=TRUE, "red"=FALSE}, "C4"={"green"=FALSE, "Yellow"=TRUE, "red"=FALSE, "Arrow"=FALSE}, "CC"={"green"=FALSE, "red"=TRUE}, "D1"={"green"=FALSE, "Yellow"=FALSE, "red"=TRUE}, "D1 2"={"green"=FALSE, "Yellow"=FALSE, "red"=TRUE}, "DD"={"green"=FALSE, "red"=TRUE}, "A1  2"={"green"=FALSE, "Yellow"=FALSE, "red"=TRUE}, "Enum_Cykl"=enum."State_3", "Enum_Stan"=enum."Mruganie", "Timer_Global"={"Numeric 3"=0, "Numeric 4"=0}, "Timer_Mruganie"={"Numeric 3"=0, "Numeric 4"=0}, "Time"=4, "Command"=enum."CheckStatus", "MessageParameters"={"Status"=enum."Light_ON", "Data"=[]}}, s=w225, f=w227) -> (s? t:f=w226:T15)
              }
            }
          }
          frame "State_4" {
            n71 = case shown="\"Czerwony\"" w230 {
              tunnel: [w235 w239 w246 w259] -> w233
              tunnel: w232 -> [w236 w240 w247 w258]
              tunnel: w231 -> [w237 w241 w243 w260]
              tunnel: w229 -> [_ _ w244 _]
              frame "Żółty" {
                n72 = Select(t=T15 {"A1 "={"green"=TRUE, "Yellow"=FALSE, "red"=FALSE}, "A3"={"green"=FALSE, "Yellow"=FALSE, "red"=TRUE, "Arrow"=FALSE}, "AAA"={"green"=TRUE, "red"=FALSE}, "B1"={"green"=FALSE, "Yellow"=FALSE, "red"=TRUE}, "B2"={"green"=FALSE, "Yellow"=FALSE, "red"=TRUE, "Arrow"=FALSE}, "BBB"={"green"=FALSE, "red"=TRUE}, "C1"={"green"=FALSE, "Yellow"=FALSE, "red"=TRUE}, "C1 2"={"green"=FALSE, "Yellow"=FALSE, "red"=TRUE}, "C4"={"green"=FALSE, "Yellow"=FALSE, "red"=TRUE, "Arrow"=FALSE}, "CC"={"green"=FALSE, "red"=TRUE}, "D1"={"green"=FALSE, "Yellow"=FALSE, "red"=TRUE}, "D1 2"={"green"=FALSE, "Yellow"=FALSE, "red"=TRUE}, "DD"={"green"=TRUE, "red"=FALSE}, "A1  2"={"green"=FALSE, "Yellow"=FALSE, "red"=TRUE}, "Enum_Cykl"=enum."State_4", "Enum_Stan"=enum."Źielony", "Timer_Global"={"Numeric 3"=0, "Numeric 4"=0}, "Timer_Mruganie"={"Numeric 3"=0, "Numeric 4"=0}, "Time"=3, "Command"=enum."CheckStatus", "MessageParameters"={"Status"=enum."Light_ON", "Data"=[]}}, s=w236, f=w237) -> (s? t:f=w235:T15)
              }
              frame "Czerwony" {
                n73 = Select(t=T15 {"A1 "={"green"=FALSE, "Yellow"=TRUE, "red"=TRUE}, "A3"={"green"=FALSE, "Yellow"=FALSE, "red"=TRUE, "Arrow"=FALSE}, "AAA"={"green"=FALSE, "red"=TRUE}, "B1"={"green"=FALSE, "Yellow"=FALSE, "red"=TRUE}, "B2"={"green"=FALSE, "Yellow"=FALSE, "red"=TRUE, "Arrow"=FALSE}, "BBB"={"green"=FALSE, "red"=TRUE}, "C1"={"green"=FALSE, "Yellow"=FALSE, "red"=TRUE}, "C1 2"={"green"=FALSE, "Yellow"=FALSE, "red"=TRUE}, "C4"={"green"=FALSE, "Yellow"=FALSE, "red"=TRUE, "Arrow"=FALSE}, "CC"={"green"=FALSE, "red"=TRUE}, "D1"={"green"=FALSE, "Yellow"=FALSE, "red"=TRUE}, "D1 2"={"green"=FALSE, "Yellow"=FALSE, "red"=TRUE}, "DD"={"green"=FALSE, "red"=TRUE}, "A1  2"={"green"=FALSE, "Yellow"=FALSE, "red"=TRUE}, "Enum_Cykl"=enum."State_4", "Enum_Stan"=enum."Żółty", "Timer_Global"={"Numeric 3"=0, "Numeric 4"=0}, "Timer_Mruganie"={"Numeric 3"=0, "Numeric 4"=0}, "Time"=3, "Command"=enum."CheckStatus", "MessageParameters"={"Status"=enum."Light_ON", "Data"=[]}}, s=w240, f=w241) -> (s? t:f=w239:T15)
              }
              frame "Mruganie" {
                n74 = case shown="True" w244 {
                  tunnel: [w248 w249] -> w245
                  tunnel: w243 -> [w248 w250]
                  frame False {
                  }
                  frame True {
                    n75 = Unbundle By Name(w250) -> ("A1.Yellow"=w255:T9, "BBB.green"=w256:bool, "DD.green"=w254:bool)
                    n76 = Not(x=w255) -> (.not. x?=w253:T9)
                    n77 = Not(x=w256) -> (.not. x?=w252:bool)
                    n78 = Not(x=w254) -> (.not. x?=w251:bool)
                    n79 = Bundle By Name(cluster=w250, "A1.Yellow"=w253, "BBB.green"=w252, "DD.green"=w251) -> (w249:T15)
                  }
                }
                n80 = Select(t=T15 {"A1 "={"green"=FALSE, "Yellow"=FALSE, "red"=TRUE}, "A3"={"green"=FALSE, "Yellow"=FALSE, "red"=TRUE, "Arrow"=FALSE}, "AAA"={"green"=TRUE, "red"=FALSE}, "B1"={"green"=FALSE, "Yellow"=FALSE, "red"=TRUE}, "B2"={"green"=FALSE, "Yellow"=FALSE, "red"=TRUE, "Arrow"=FALSE}, "BBB"={"green"=FALSE, "red"=TRUE}, "C1"={"green"=FALSE, "Yellow"=FALSE, "red"=TRUE}, "C1 2"={"green"=FALSE, "Yellow"=FALSE, "red"=TRUE}, "C4"={"green"=FALSE, "Yellow"=FALSE, "red"=TRUE, "Arrow"=FALSE}, "CC"={"green"=FALSE, "red"=TRUE}, "D1"={"green"=FALSE, "Yellow"=FALSE, "red"=TRUE}, "D1 2"={"green"=FALSE, "Yellow"=FALSE, "red"=TRUE}, "DD"={"green"=TRUE, "red"=FALSE}, "A1  2"={"green"=FALSE, "Yellow"=FALSE, "red"=TRUE}, "Enum_Cykl"=enum."State_1", "Enum_Stan"=enum."Czerwony", "Timer_Global"={"Numeric 3"=0, "Numeric 4"=0}, "Timer_Mruganie"={"Numeric 3"=0, "Numeric 4"=0}, "Time"=1, "Command"=enum."CheckStatus", "MessageParameters"={"Status"=enum."Light_ON", "Data"=[]}}, s=w247, f=w245) -> (s? t:f=w246:T15)
              }
              frame "Źielony" {
                n81 = Select(t=T15 {"A1 "={"green"=FALSE, "Yellow"=TRUE, "red"=FALSE}, "A3"={"green"=FALSE, "Yellow"=FALSE, "red"=TRUE, "Arrow"=FALSE}, "AAA"={"green"=TRUE, "red"=FALSE}, "B1"={"green"=FALSE, "Yellow"=FALSE, "red"=TRUE}, "B2"={"green"=FALSE, "Yellow"=FALSE, "red"=TRUE, "Arrow"=FALSE}, "BBB"={"green"=TRUE, "red"=FALSE}, "C1"={"green"=FALSE, "Yellow"=FALSE, "red"=TRUE}, "C1 2"={"green"=FALSE, "Yellow"=FALSE, "red"=TRUE}, "C4"={"green"=FALSE, "Yellow"=FALSE, "red"=TRUE, "Arrow"=FALSE}, "CC"={"green"=FALSE, "red"=TRUE}, "D1"={"green"=FALSE, "Yellow"=FALSE, "red"=TRUE}, "D1 2"={"green"=FALSE, "Yellow"=FALSE, "red"=TRUE}, "DD"={"green"=FALSE, "red"=TRUE}, "A1  2"={"green"=FALSE, "Yellow"=FALSE, "red"=TRUE}, "Enum_Cykl"=enum."State_4", "Enum_Stan"=enum."Mruganie", "Timer_Global"={"Numeric 3"=0, "Numeric 4"=0}, "Timer_Mruganie"={"Numeric 3"=0, "Numeric 4"=0}, "Time"=3, "Command"=enum."CheckStatus", "MessageParameters"={"Status"=enum."Light_ON", "Data"=[]}}, s=w258, f=w260) -> (s? t:f=w259:T15)
              }
            }
          }
          frame "Breakdown" {
            n82 = case shown="True" w265 {
              tunnel: [T15 {"A1 "={"green"=FALSE, "Yellow"=TRUE, "red"=FALSE}, "A3"={"green"=FALSE, "Yellow"=TRUE, "red"=FALSE, "Arrow"=FALSE}, "AAA"={"green"=FALSE, "red"=FALSE}, "B1"={"green"=FALSE, "Yellow"=TRUE, "red"=FALSE}, "B2"={"green"=FALSE, "Yellow"=TRUE, "red"=FALSE, "Arrow"=FALSE}, "BBB"={"green"=FALSE, "red"=FALSE}, "C1"={"green"=FALSE, "Yellow"=TRUE, "red"=FALSE}, "C1 2"={"green"=FALSE, "Yellow"=TRUE, "red"=FALSE}, "C4"={"green"=FALSE, "Yellow"=TRUE, "red"=FALSE, "Arrow"=FALSE}, "CC"={"green"=FALSE, "red"=FALSE}, "D1"={"green"=FALSE, "Yellow"=TRUE, "red"=FALSE}, "D1 2"={"green"=FALSE, "Yellow"=TRUE, "red"=FALSE}, "DD"={"green"=FALSE, "red"=FALSE}, "A1  2"={"green"=FALSE, "Yellow"=TRUE, "red"=FALSE}, "Enum_Cykl"=enum."Breakdown", "Enum_Stan"=enum."Czerwony", "Timer_Global"={"Numeric 3"=0, "Numeric 4"=0}, "Timer_Mruganie"={"Numeric 3"=0, "Numeric 4"=0}, "Time"=1, "Command"=enum."CheckStatus", "MessageParameters"={"Status"=enum."Light_ON", "Data"=[]}} T15 {"A1 "={"green"=FALSE, "Yellow"=FALSE, "red"=FALSE}, "A3"={"green"=FALSE, "Yellow"=FALSE, "red"=FALSE, "Arrow"=FALSE}, "AAA"={"green"=FALSE, "red"=FALSE}, "B1"={"green"=FALSE, "Yellow"=FALSE, "red"=FALSE}, "B2"={"green"=FALSE, "Yellow"=FALSE, "red"=FALSE, "Arrow"=FALSE}, "BBB"={"green"=FALSE, "red"=FALSE}, "C1"={"green"=FALSE, "Yellow"=FALSE, "red"=FALSE}, "C1 2"={"green"=FALSE, "Yellow"=FALSE, "red"=FALSE}, "C4"={"green"=FALSE, "Yellow"=FALSE, "red"=FALSE, "Arrow"=FALSE}, "CC"={"green"=FALSE, "red"=FALSE}, "D1"={"green"=FALSE, "Yellow"=FALSE, "red"=FALSE}, "D1 2"={"green"=FALSE, "Yellow"=FALSE, "red"=FALSE}, "DD"={"green"=FALSE, "red"=FALSE}, "A1  2"={"green"=FALSE, "Yellow"=FALSE, "red"=FALSE}, "Enum_Cykl"=enum."Breakdown", "Enum_Stan"=enum."Czerwony", "Timer_Global"={"Numeric 3"=0, "Numeric 4"=0}, "Timer_Mruganie"={"Numeric 3"=0, "Numeric 4"=0}, "Time"=1, "Command"=enum."CheckStatus", "MessageParameters"={"Status"=enum."Light_ON", "Data"=[]}}] -> w262
              frame False {
              }
              frame True {
              }
            }
            n83 = Select(t=T15 {"A1 "={"green"=FALSE, "Yellow"=TRUE, "red"=TRUE}, "A3"={"green"=FALSE, "Yellow"=FALSE, "red"=TRUE, "Arrow"=FALSE}, "AAA"={"green"=FALSE, "red"=TRUE}, "B1"={"green"=FALSE, "Yellow"=FALSE, "red"=TRUE}, "B2"={"green"=FALSE, "Yellow"=FALSE, "red"=TRUE, "Arrow"=FALSE}, "BBB"={"green"=FALSE, "red"=TRUE}, "C1"={"green"=FALSE, "Yellow"=FALSE, "red"=TRUE}, "C1 2"={"green"=FALSE, "Yellow"=FALSE, "red"=TRUE}, "C4"={"green"=FALSE, "Yellow"=FALSE, "red"=TRUE, "Arrow"=FALSE}, "CC"={"green"=FALSE, "red"=TRUE}, "D1"={"green"=FALSE, "Yellow"=FALSE, "red"=TRUE}, "D1 2"={"green"=FALSE, "Yellow"=FALSE, "red"=TRUE}, "DD"={"green"=FALSE, "red"=TRUE}, "A1  2"={"green"=FALSE, "Yellow"=FALSE, "red"=TRUE}, "Enum_Cykl"=enum."State_4", "Enum_Stan"=enum."Żółty", "Timer_Global"={"Numeric 3"=0, "Numeric 4"=0}, "Timer_Mruganie"={"Numeric 3"=0, "Numeric 4"=0}, "Time"=3, "Command"=enum."CheckStatus", "MessageParameters"={"Status"=enum."Light_ON", "Data"=[]}}, s="Boolean", f=w262) -> (s? t:f=w263:T15)
          }
        }
        n84 = Bundle By Name(cluster=w109, "Timer_Global"=w107, "Timer_Mruganie"=w82) -> (w108:T15)
      }
    }
    n85 = Select(t=Enum_state."Exit", s="Stop", f=w7) -> (s? t:f=w11:T23)
  }
